vi "Configure Module Dialog.vi"(8 "error in (no error)":errorcluster, 9 "Possible Modules":string[](array[string]), 10 "Existing Modules":string[](array[string]), 11 "Source":string) -> (0 "error out":errorcluster, 1 "Canceled?":bool, 2 "New Module Path":string)   [LabVIEW 2017, in "Routing and Faulting System Explorer.lvlib"]
uses:
  Routing and Faulting System Explorer.lvlib
  <vilib>/event_ctls.llb/lveventtype.ctl
  Shared/UI Common/UI Common.lvlib
panel:
  in  "New Module Path":u16(ring) items=["Mod0", "Mod1", "Mod2"]
  in  "Cancel Button":bool
  in  "OK Button":bool
  out "Description":string
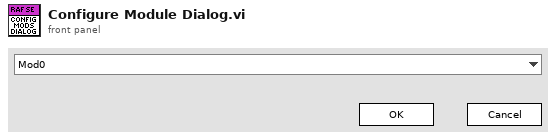
[diagram p1: front panel]
types:
  T1 = typedef "lveventtype.ctl" = enum32{"Null", "Timeout", "Annotation Menu Selection", "Annotation Menu Selection?", "App Instance Close", "App Instance Close?", "Autoscale Range Change", "Bookmark Info Change", "Cell Edit", "Cell Edit?", "Cursor Grab", "Cursor Grab?", "Cursor Menu Selection", "Cursor Menu Selection?", "Cursor Move", "Cursor Release", "Data Change", "Direction Change", "Display State Change", "Drag Ended", "Drag Enter", "Drag Leave", "Drag Over", "Drag Source Update", "Drag Starting", "Drag Starting?", "Drop", "Exec State Change", "Key Down", "Key Down?", "Key Repeat", "Key Repeat?", "Key Up", "Listbox Double Click", "Menu Activation?", "Menu Selection (App)", "Menu Selection? (App)", "Menu Selection (User)", "Mouse Down", "Mouse Down?", "Mouse Enter", "Mouse Leave", "Mouse Move", "Mouse Up", "Mouse Wheel", "NI Security User Change (App)", "Pane Size", "Panel Close", "Panel Close?", "Panel Resize", "Plot Attribute Change", "Scale Range Change", "Shortcut Menu Activation?", "Shortcut Menu Selection (App)", "Shortcut Menu Selection? (App)", "Shortcut Menu Selection (User)", "Tree Double Click", "Tree Drag", "Tree Drag?", "Tree Drop", "Tree Drop?", "Tree Item Close", "Tree Item Close?", "Tree Item Open", "Tree Item Open?", "User Event", "Value Change"}
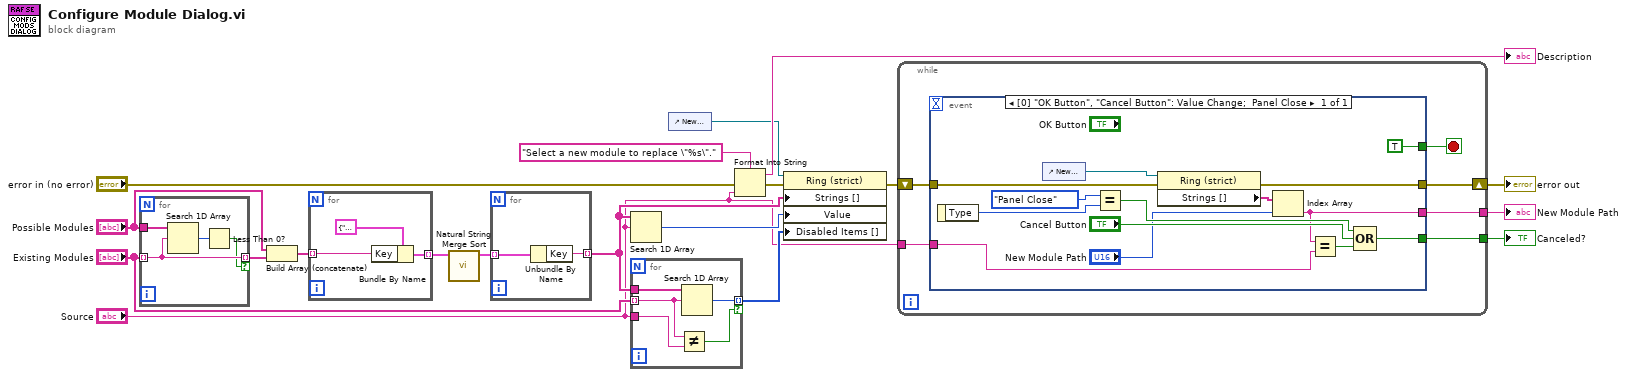
[diagram p0: block diagram]
diagram:
  n1 = for {
    tunnel: "Existing Modules" -> [w21] mode=indexing
    tunnel: "Possible Modules" -> [w23]
    tunnel: [w21] -> w4 mode=indexing if=w20
    n2 = Search 1D Array(1D array=w23, element=w21) -> (index of element=w22:i32)  [unwired: 1 in]
    n3 = Less Than 0?(x=w22) -> (x < 0?=w20:bool)
  }
  n4 = Build Array (concatenate)("Possible Modules", w4) -> (w8:string[])
  n5 = for {
    tunnel: w8 -> [w25] mode=indexing
    tunnel: [w24] -> w7 mode=indexing
    n6 = Bundle By Name(cluster=cluster{"Key":string, "Value":variant} {"Key"="", "Value"=variant} ("Cluster"), "Key"=w25) -> (w24:cluster{"Key":string, "Value":variant})
  }
  n7 = call "Natural String Merge Sort.vi"("Array in"=w7) -> ("Array out"=w6:cluster{"Key":string, "Value":variant}[])  [unwired: 10 in]
  n8 = for {
    tunnel: w6 -> [w28] mode=indexing
    tunnel: [w27] -> w5 mode=indexing
    n9 = Unbundle By Name(w28) -> ("Key"=w27:string)
  }
  n10 = Search 1D Array(1D array=w5, element="Source") -> (index of element=w11:i32)  [unwired: 1 in]
  n11 = for {
    tunnel: w5 -> [w33]
    tunnel: "Existing Modules" -> [w31] mode=indexing
    tunnel: [w32] -> w3 mode=indexing if=w29
    tunnel: "Source" -> [w30]
    n12 = Not Equal?(x=w31, y=w30) -> (x != y?=w29:bool)
    n13 = Search 1D Array(1D array=w33, element=w31) -> (index of element=w32:i32)  [unwired: 1 in]
  }
  n14 = control-ref of="New Module Path"() -> (w13:refnum<vi>)
  n15 = Format Into String(format string="Select a new module to replace \"%s\"." ("initial string"), error in="error in (no error)", "Source") -> (resulting string=→"Description":string, error out=w9:errorcluster)  [unwired: 1 in]
  n16 = property class="Ring (strict)"(reference=w13, error in=w9, "Strings []"=w5, "Value"=w11, "Disabled Items []"=w3) -> (error out=w10:errorcluster)  [unwired: 1 out]
  n17 = while {
    tunnel: [w38] -> w16
    tunnel: [w37] -> w14
    shift-right: [w34] -> w15
    shift-left: w10 -> [w35]
    tunnel: "Source" -> [w36]
    stop <- w39 stop-if-true
    n18 = event shown="[0] \"OK Button\", \"Cancel Button\": Value Change;  Panel Close" {
      selector: _ -> [_]
      dyn-events: _ -> [_]
      timeout: _ -> [_]
      tunnel: [TRUE] -> w39
      tunnel: [w48] -> w38
      tunnel: [w42] -> w37
      tunnel: w36 -> [w46]
      tunnel: w35 -> [w41]
      tunnel: [w40] -> w34
      event "OK Button", "Cancel Button": Value Change; Panel Close {
        n19 = event-data() -> ("Type"=w53:T1)  [unwired: 1 in]
        n20 = control-ref of="New Module Path"() -> (w45:refnum<vi>)
        n21 = Equal?(x=lveventtype."Panel Close" ("Type"), y=w53) -> (x = y?=w51:bool)
        n22 = property class="Ring (strict)"(reference=w45, error in=w41) -> (error out=w40:errorcluster, "Strings []"=w44:string[])  [unwired: 1 out]
        n23 = Index Array(array=w44, index="New Module Path") -> (element=w42:string)
        n24 = Equal?(x=w42, y=w46) -> (x = y?=w47:bool)
        n25 = Compound Arithmetic op=OR(w51, "Cancel Button", w47) -> (w48:bool)
      }
    }
  }
  "error out" <- w15
  "Canceled?" <- w16
  "New Module Path" <- w14
